vi "Set_Do_Array.vi"(8 "error in (no error)":errorcluster, 10 "DOs":bool[](array[boolean]), 11 "reference in":refnum<class "FPGA_Interface.lvclass">) -> (0 "error out":errorcluster, 3 "reference out":refnum<class "FPGA_Interface.lvclass">)   [LabVIEW 2019, in "FPGA_Interface.lvclass"]
uses:
  FPGA_Interface.lvclass
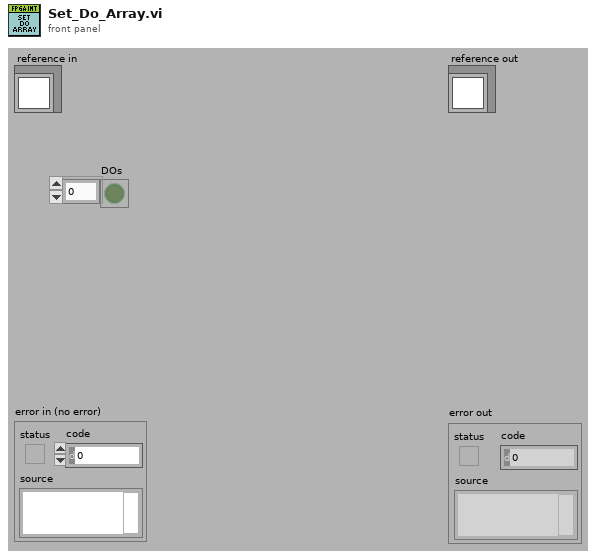
[diagram p1: front panel]
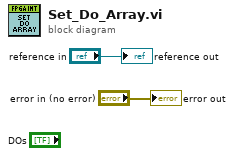
[diagram p0: block diagram]
diagram:
  "error out" <- "error in (no error)"
  "reference out" <- "reference in"
